vi "Find all Bonds in Structure.vi"(10 "Max Bond Length":dbl, 11 "Structure":T2={"Structure ID"="Batch3_1", "Lattice vector a"=[6.48, 0.0, 0.0], "Lattice vector b"=[0.0, 6.48, 0.0], "Lattice vector c"=[0.0, 0.0, 31.06], "Atoms Array"=[{"Atom Name"="Cd", "Positions (Direct)"=[[0.0, 0.0, 0.00272], [0.5, 0.5, 0.00272], [0.5, 0.0, 0.110479], [0.0, 0.5, 0.110479], [0.0, 0.0, 0.218487], [0.5, 0.5, 0.218487], [0.5, 0.0, 0.32654], [0.0, 0.5, 0.32654], [0.25, 0.25, 0.427635], [0.75, 0.75, 0.427635], [0.0, 0.0, 0.570345], [0.5, 0.5, 0.570345], [0.5, 0.0, 0.679049], [0.0, 0.5, 0.679049], [0.0, 0.0, 0.786972], [0.5, 0.5, 0.786972], [0.5, 0.0, 0.894944], [0.0, 0.5, 0.894944]], "Positions (Cartesian)"=[[0.0, 0.0, 0.08448320000000001], [3.24, 3.24, 0.08448320000000001], [3.24, 0.0, 3.4314777399999996], [0.0, 3.24, 3.4314777399999996], [0.0, 0.0, 6.7862062199999995], [3.24, 3.24, 6.7862062199999995], [3.24, 0.0, 10.142332399999999], [0.0, 3.24, 10.142332399999999], [1.62, 1.62, 13.282343099999999], [4.86, 4.86, 13.282343099999999], [0.0, 0.0, 17.7149157], [3.24, 3.24, 17.7149157], [3.24, 0.0, 21.09126194], [0.0, 3.24, 21.09126194], [0.0, 0.0, 24.44335032], [3.24, 3.24, 24.44335032], [3.24, 0.0, 27.796960639999998], [0.0, 3.24, 27.796960639999998]]}, {"Atom Name"="Te", "Positions (Direct)"=[[0.25, 0.25, 0.055996], [0.75, 0.75, 0.055996], [0.75, 0.25, 0.163889], [0.25, 0.75, 0.163889], [0.25, 0.25, 0.271952], [0.75, 0.75, 0.271952], [0.75, 0.25, 0.383704], [0.25, 0.75, 0.383704], [0.0, 0.0, 0.483915], [0.5, 0.5, 0.483915], [0.25, 0.25, 0.623906], [0.75, 0.75, 0.623906], [0.75, 0.25, 0.732362], [0.25, 0.75, 0.732362], [0.25, 0.25, 0.840344], [0.75, 0.75, 0.840344], [0.75, 0.25, 0.948333], [0.25, 0.75, 0.948333]], "Positions (Cartesian)"=[[1.62, 1.62, 1.73923576], [4.86, 4.86, 1.73923576], [4.86, 1.62, 5.09039234], [1.62, 4.86, 5.09039234], [1.62, 1.62, 8.44682912], [4.86, 4.86, 8.44682912], [4.86, 1.62, 11.91784624], [1.62, 4.86, 11.91784624], [0.0, 0.0, 15.030399899999999], [3.24, 3.24, 15.030399899999999], [1.62, 1.62, 19.37852036], [4.86, 4.86, 19.37852036], [4.86, 1.62, 22.747163719999996], [1.62, 4.86, 22.747163719999996], [1.62, 1.62, 26.10108464], [4.86, 4.86, 26.10108464], [4.86, 1.62, 29.45522298], [1.62, 4.86, 29.45522298]]}], "# of atoms"=36}) -> (3 "Bonds":T1(array[cluster]))   [LabVIEW 2010]
uses:
  <vilib>/Analysis/_algsub.llb/Real Vector Norm.vi
  <vilib>/Analysis/NI_AALPro.lvlib
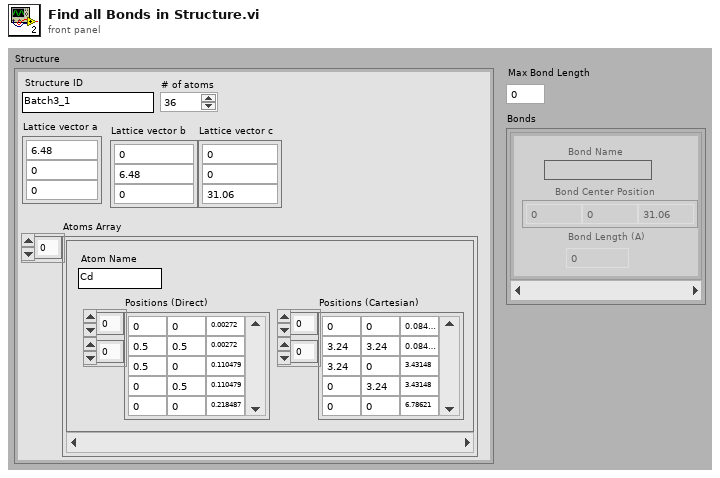
[diagram p1: front panel]
types:
  T1 = cluster{"Bond Name":string, "Bond Center Position":dbl[], "Bond Length (A)":dbl}[]
  T2 = cluster{"Structure ID":string, "Lattice vector a":dbl[], "Lattice vector b":dbl[], "Lattice vector c":dbl[], "Atoms Array":cluster{"Atom Name":string, "Positions (Direct)":dbl[][], "Positions (Cartesian)":dbl[][]}[], "# of atoms":i32}
  T3 = cluster{"Atom Name":string, i32, "Positions (Cartesian)":dbl[]}[]
  T4 = cluster{"Atom Name":string, "Positions (Direct)":dbl[][], "Positions (Cartesian)":dbl[][]}[]
  T5 = cluster{"Atom Name":string, i32, "Positions (Cartesian)":dbl[]}
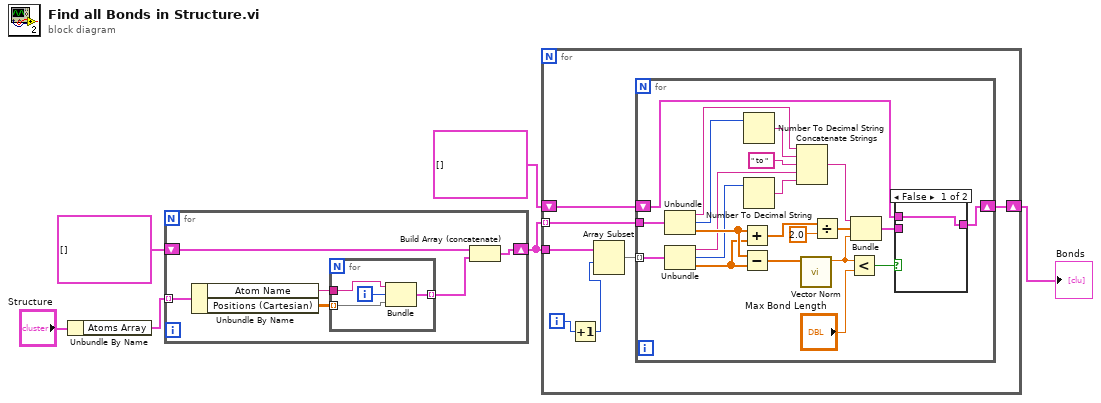
[diagram p0: block diagram]
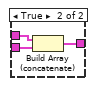
[diagram p2: hidden frame]
diagram:
  n1 = Unbundle By Name("Structure") -> ("Atoms Array"=w5:T4)
  n2 = for {
    tunnel: w5 -> [w12] mode=indexing
    shift-right: [w8] -> w3
    shift-left: T3 [] -> [w7]
    n3 = Unbundle By Name(w12) -> ("Atom Name"=w9:string, "Positions (Cartesian)"=w11:dbl[][])
    n4 = for {
      tunnel: w11 -> [w16] mode=indexing
      tunnel: [w15] -> w10 mode=indexing
      tunnel: w9 -> [w14]
      i -> [w13]
      n5 = Bundle("Atom Name"=w14, w13, "Positions (Cartesian)"=w16) -> (w15:T5)  [unwired: 1 in]
    }
    n6 = Build Array (concatenate)(w7, w10) -> (w8:T3)
  }
  n7 = for {
    tunnel: w3 -> [w23] mode=indexing
    tunnel: w3 -> [w22]
    shift-right: [w20] -> w1
    shift-left: cluster{string, dbl[], "norm":dbl}[] [] -> [w19]
    i -> [w18]
    n8 = Increment(x=w18) -> (x+1=w17:i32)
    n9 = Array Subset(array=w22, index=w17) -> (w21:T3)  [unwired: 1 in]
    n10 = for {
      tunnel: w23 -> [w45]
      tunnel: w21 -> [w44] mode=indexing
      shift-right: [w25] -> w20
      shift-left: w19 -> [w24]
      n11 = Unbundle(w45) -> ("Atom Name"=w37:string, w36:i32, "Positions (Cartesian)"=w39:dbl[])
      n12 = Unbundle(w44) -> ("Atom Name"=w33:string, w32:i32, "Positions (Cartesian)"=w38:dbl[])
      n13 = Add(x=w39, y=w38) -> (x+y=w41:dbl[])
      n14 = Subtract(x=w39, y=w38) -> (x-y=w43:dbl[])
      n15 = Number To Decimal String(number=w36) -> (decimal integer string=w35:string)  [unwired: 1 in]
      n16 = Number To Decimal String(number=w32) -> (decimal integer string=w31:string)  [unwired: 1 in]
      n17 = Concatenate Strings(w37, w35, " to " ("string"), w33, w31) -> (w30:string)
      n18 = call-poly <vilib>:"Vector Norm.vi"("Input Vector"=w43) -> ("norm"=w27:dbl)  [unwired: 9 in, 1 out]
      n19 = Divide(x=w41, y=2.0) -> (x/y=w40:dbl[])
      n20 = Less?(x=w27, y="Max Bond Length") -> (x < y?=w28:bool)
      n21 = Bundle(w30, w40, "norm"=w27) -> (w29:cluster{string, dbl[], "norm":dbl})  [unwired: 1 in]
      n22 = case shown="False" w28 {
        tunnel: w29 -> [_ w49]
        tunnel: [w46 w48] -> w25
        tunnel: w24 -> [w46 w47]
        frame False {
        }
        frame True {
          n23 = Build Array (concatenate)(w47, w49) -> (w48:cluster{string, dbl[], "norm":dbl}[])
        }
      }
    }
  }
  "Bonds" <- w1
